vi "direction_channel_fgv.vi"(7 "Index":i32, 8 "error in (no error)":errorcluster, 9 "aData Out":dbl[][](array[numeric]), 11 "op":T1) -> (0 "error out":errorcluster, 3 "direction":i64)   [LabVIEW 2025, in "LabJackEKG.lvlib"]
uses:
  LabJackEKG.lvlib
  Typedefs/DirectionFgvOperation.ctl
panel:
  in  "threshold":i64=4
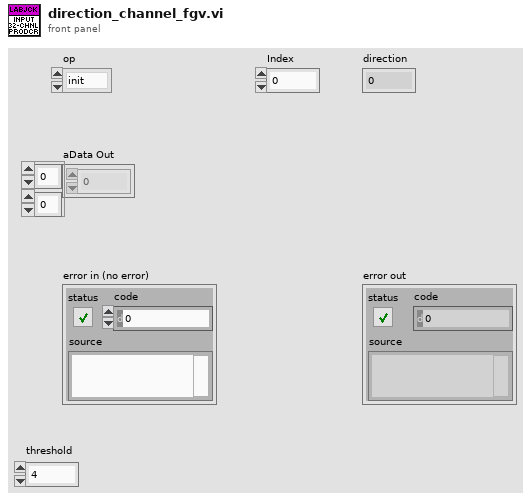
[diagram p1: front panel]
types:
  T1 = typedef "LabJackEKG.lvlib/DirectionFgvOperation.ctl" = enum16{"init", "process", "get"}
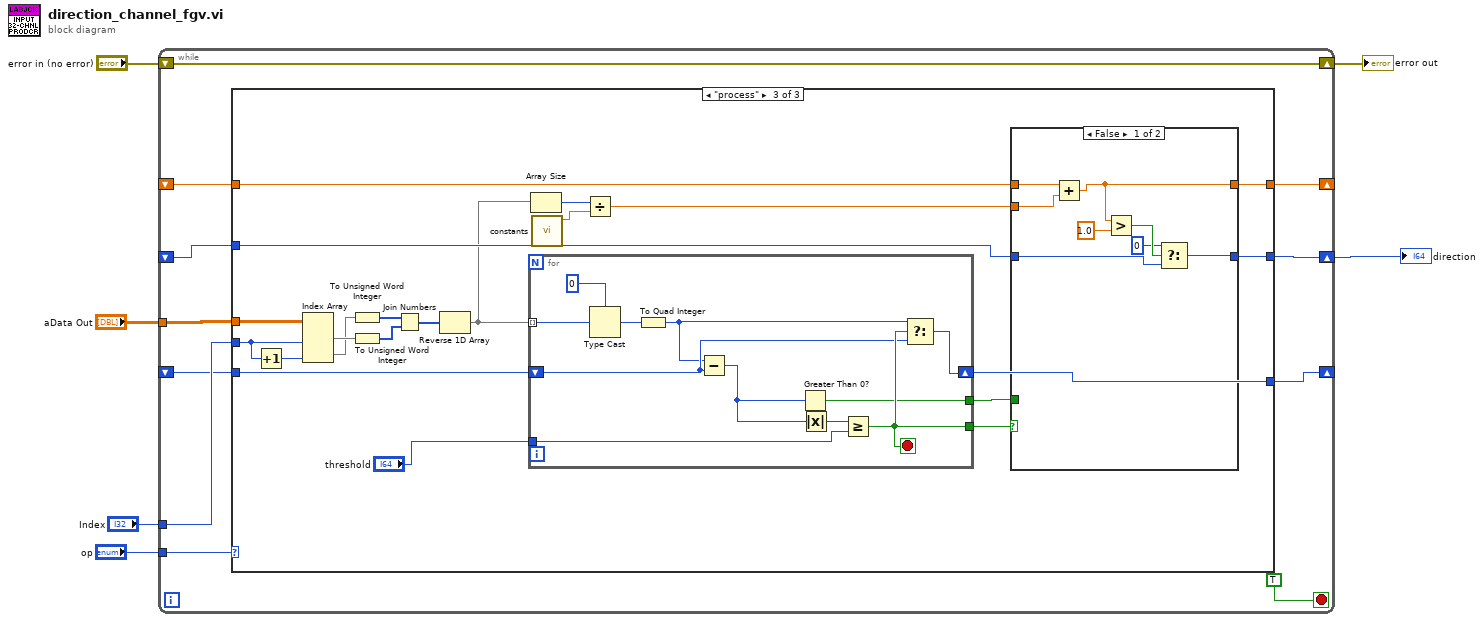
[diagram p0: block diagram]
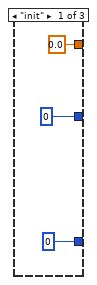
[diagram p2: hidden frame]
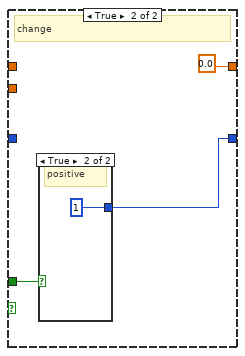
[diagram p4: hidden frame]
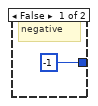
[diagram p5: hidden frame]
diagram:
  n1 = while {
    tunnel: "aData Out" -> [w17]
    tunnel: "Index" -> [w16]
    shift-right: [w9] -> w6
    shift-left: "error in (no error)" -> [w9]
    tunnel: "op" -> [w15]
    shift-right: [w11] -> w1
    shift-left: _ -> [w14]
    shift-right: [w12] -> _
    shift-left: _ -> [w13]
    shift-right: [w8] -> _
    shift-left: _ -> [w7]
    stop <- TRUE stop-if-true
    n2 = case shown="\"process\"" w15 {
      tunnel: w17 -> [_ _ w44]
      tunnel: w16 -> [_ _ w41]
      tunnel: w14 -> [_ w23 w32]
      tunnel: w13 -> [_ w22 w36]
      tunnel: [i64 0 w22 w34] -> w12
      tunnel: [i64 0 w23 w33] -> w11
      tunnel: [0.0 w21 w26] -> w8
      tunnel: w7 -> [_ w21 w25]
      frame "init" {
      }
      frame "get" {
      }
      frame "process" {
        n3 = Increment(x=w41) -> (x+1=w40:i32)
        n4 = Index Array(array=w44, index (col) #1=w41, index (col) #2=w40) -> (element #1=w43:dbl[], element #2=w42:dbl[])  [unwired: 2 in]
        n5 = To Unsigned Word Integer(number=w42) -> (unsigned 16bit integer=w38:u16[])
        n6 = To Unsigned Word Integer(number=w43) -> (unsigned 16bit integer=w39:u16[])
        n7 = Join Numbers(hi=w38, lo=w39) -> ((hi.lo)=w37:u32[])
        n8 = Reverse 1D Array(array=w37) -> (reversed array=w30:u32[])
        n9 = for {
          tunnel: w30 -> [w67] mode=indexing
          shift-right: [w60] -> w34
          shift-left: w36 -> [w63]
          tunnel: [w64] -> w35
          tunnel: [w61] -> w31
          tunnel: "threshold" -> [w58]
          stop <- w64 stop-if-true
          n10 = Type Cast(type=0, x=w67) -> (*(type *) &x=w68:i32)
          n11 = To Quad Integer(1:w68) -> (0:w59:i64)
          n12 = Subtract(x=w59, y=w63) -> (x-y=w62:i64)
          n13 = Greater Than 0?(x=w62) -> (x > 0?=w61:bool)
          n14 = Absolute Value(x=w62) -> (abs(x)=w65:i64)
          n15 = Greater Or Equal?(x=w65, y=w58) -> (x >= y?=w64:bool)
          n16 = Select(t=w59, s=w64, f=w63) -> (s? t:f=w60:i64)
        }
        n17 = Array Size(array=w30) -> (size(s)=w29:i32)
        n18 = call "constants.vi"() -> ("Sampling Frequency [Hz]"=w28:dbl)  [unwired: 10 in, 1 out]
        n19 = Divide(x=w29, y=w28) -> (x/y=w27:dbl)
        n20 = case shown="False" w35 {
          tunnel: [w45 w55] -> w33
          tunnel: w32 -> [w48 _]
          tunnel: w31 -> [_ w54]
          tunnel: w27 -> [w51 _]
          tunnel: [w50 0.0] -> w26
          tunnel: w25 -> [w52 _]
          frame False {
            n21 = Add(x=w52, y=w51) -> (x+y=w50:dbl)
            n22 = Greater?(x=w50, y=1.0) -> (0:w47:bool)
            n23 = Select(t=i64 0, s=w47, f=w48) -> (s? t:f=w45:i64)
          }
          frame True {
            # "change"
            n24 = case shown="True" w54 {
              tunnel: [i64 -1 i64 1] -> w55
              frame False {
                # "negative"
              }
              frame True {
                # "positive"
              }
            }
          }
        }
      }
    }
  }
  "error out" <- w6
  "direction" <- w1
